vi "wd_create (WFM).vi"(7 "WFM":waveform(dbl), 8 "error in (no error)":errorcluster, 9 "data type":T1, 11 "meta in":T2={"TargetFile"=path "", "StreamMode"=enum."File", "Append?"=FALSE, "ChunkSize"=0, "TimeColumnMode"=enum."Empty", "TimestampFormat"="", "AbsoluteTime?"=FALSE, "FileAttribute "={"Creator"="", "Title"="", "SheetName"=""}, "Column"=[], "FileRef"=refnum, "MemoryRef"=[], "RecordInfo"=[], " ChannelPreviousInfo"=[], "ChannelFirstRecord"=[], "PredefinedFormattedValueLength"=20, "DiskTemplate"={"XMLRef"=[refnum, refnum, refnum, refnum, refnum, refnum], "ZipPath"=path "", "MetaFile"={"Ref"=refnum, "NextRow"=0, "NextPosition"=0, "Block"=[]}, "TempFolder"=path ""}}) -> (0 "error out":errorcluster, 3 "meta out":T2={"TargetFile"=path "", "StreamMode"=enum."File", "Append?"=FALSE, "ChunkSize"=0, "TimeColumnMode"=enum."Empty", "TimestampFormat"="", "AbsoluteTime?"=FALSE, "FileAttribute "={"Creator"="", "Title"="", "SheetName"=""}, "Column"=[], "FileRef"=refnum, "MemoryRef"=[], "RecordInfo"=[], " ChannelPreviousInfo"=[], "ChannelFirstRecord"=[], "PredefinedFormattedValueLength"=20, "DiskTemplate"={"XMLRef"=[refnum, refnum, refnum, refnum, refnum, refnum], "ZipPath"=path "", "MetaFile"={"Ref"=refnum, "NextRow"=0, "NextPosition"=0, "Block"=[]}, "TempFolder"=path ""}})   [LabVIEW 2020, in "NI_ExcelFile.lvlib"]
uses:
  <vilib>/express/express shared/NI_ExcelFile/NI_ExcelFile.lvlib
  <vilib>/express/express shared/NI_ExcelFile/Ctrls/MainData.ctl
  <vilib>/express/express shared/NI_ExcelFile/Ctrls/StreamMode.ctl
  <vilib>/express/express shared/NI_ExcelFile/Ctrls/TimeColumnMode.ctl
  <vilib>/express/express shared/NI_ExcelFile/Ctrls/FileAttribute.ctl
  <vilib>/express/express shared/NI_ExcelFile/Ctrls/Columns.ctl
  <vilib>/express/express shared/NI_ExcelFile/Ctrls/ColumnInfo.ctl
  <vilib>/express/express shared/NI_ExcelFile/Ctrls/DataType.ctl
  <vilib>/express/express shared/NI_ExcelFile/Ctrls/wd_recordInfo.ctl
  <vilib>/express/express shared/NI_ExcelFile/Ctrls/disk_TemplateFile.ctl
  <vilib>/express/express shared/NI_ExcelFile/Ctrls/meta_file.ctl
  <vilib>/express/express shared/NI_ExcelFile/Ctrls/meta_Block.ctl
  <vilib>/express/express shared/NI_ExcelFile/Ctrls/meta_BlockType.ctl
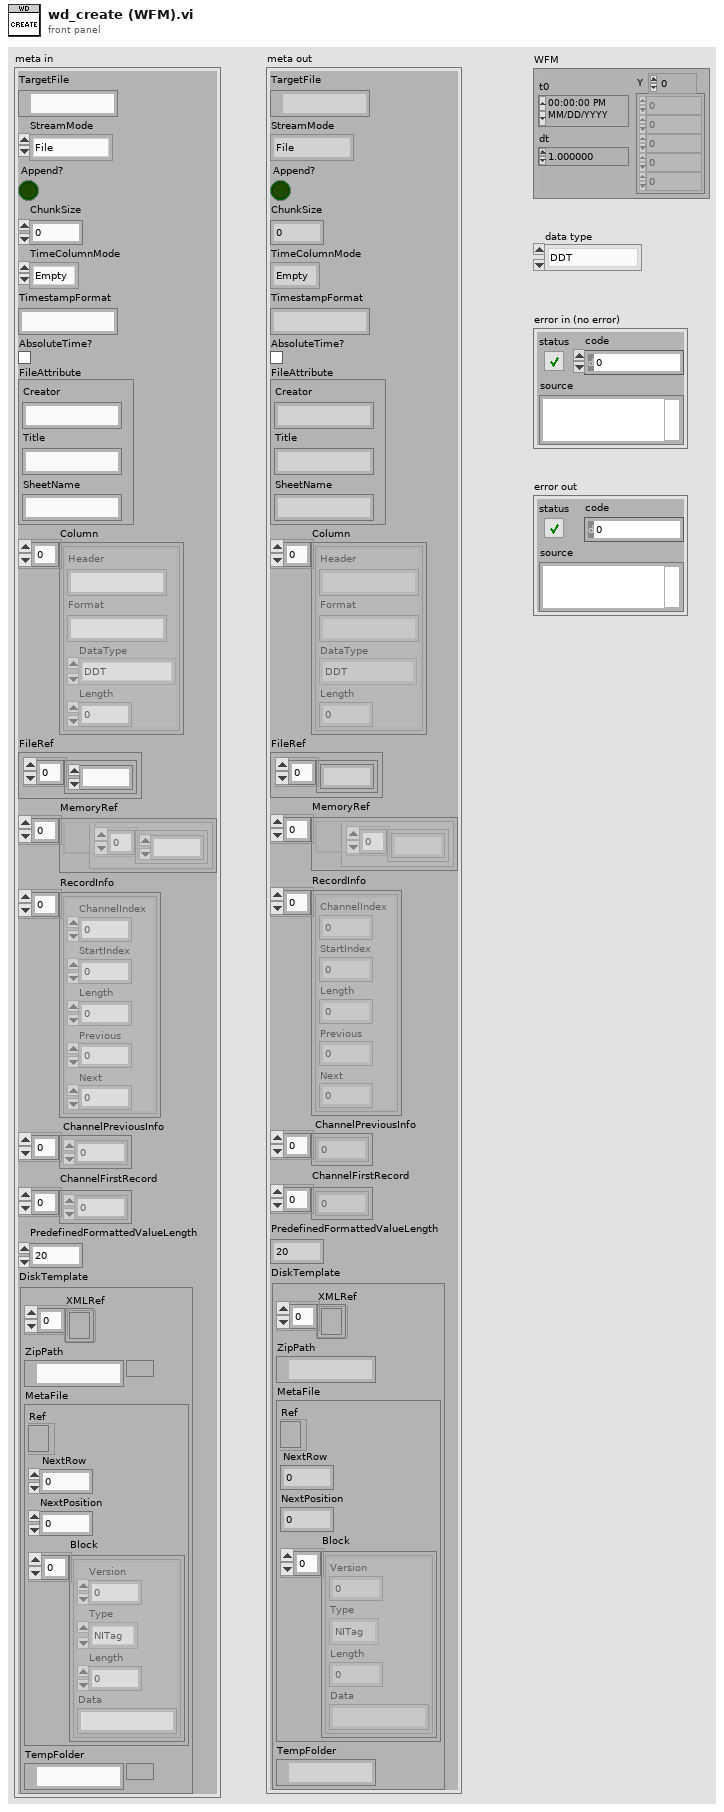
[diagram p1: front panel]
types:
  T1 = typedef "NI_ExcelFile.lvlib/DataType.ctl" = enum16{"DDT", "WFM", "Array of STR", "Array of DBL", "Array of I8", "Array of I16", "Array of I32", "Array of I64", "Array of SGL", "Array of U8", "Array of U16", "Array of U32", "Array of U64", "Array of Time"}
  T2 = typedef "NI_ExcelFile.lvlib/MainData.ctl" = cluster{"TargetFile":path, "StreamMode":T3, "Append?":bool, "ChunkSize":u64, "TimeColumnMode":T4, "TimestampFormat":string, "AbsoluteTime?":bool, "FileAttribute ":T5, "Column":T6, "FileRef":refnum<k1>, "MemoryRef":refnum<data-value>[], "RecordInfo":T8[], " ChannelPreviousInfo":u32[], "ChannelFirstRecord":u32[], "PredefinedFormattedValueLength":i64, "DiskTemplate":T9}
  T3 = typedef "NI_ExcelFile.lvlib/StreamMode.ctl" = enum16{"File", "Memory"}
  T4 = typedef "NI_ExcelFile.lvlib/TimeColumnMode.ctl" = enum16{"Empty", "OnePerCh", "One"}
  T5 = typedef "NI_ExcelFile.lvlib/FileAttribute.ctl" = cluster{"Creator":string, "Title":string, "SheetName":string}
  T6 = typedef "NI_ExcelFile.lvlib/Columns.ctl" = T7[]
  T7 = typedef "NI_ExcelFile.lvlib/ColumnInfo.ctl" = cluster{"Header":string, "Format":string, "DataType":T1, "Length":u64}
  T8 = typedef "NI_ExcelFile.lvlib/wd_recordInfo.ctl" = cluster{"ChannelIndex":u32, "StartIndex":u64, "Length":u64, "Previous":i32, "Next":i32}
  T9 = typedef "NI_ExcelFile.lvlib/disk_TemplateFile.ctl" = cluster{"XMLRef":refnum<file>[], "ZipPath":path, "MetaFile":T10, "TempFolder":path}
  T10 = typedef "NI_ExcelFile.lvlib/meta_file.ctl" = cluster{"Ref":refnum<file>, "NextRow":i32, "NextPosition":i64, "Block":T11[]}
  T11 = typedef "NI_ExcelFile.lvlib/meta_Block.ctl" = cluster{"Version":u16, "Type":T12, "Length":i32, "Data":string}
  T12 = typedef "NI_ExcelFile.lvlib/meta_BlockType.ctl" = enum16{"NITag", "File", "Column"}
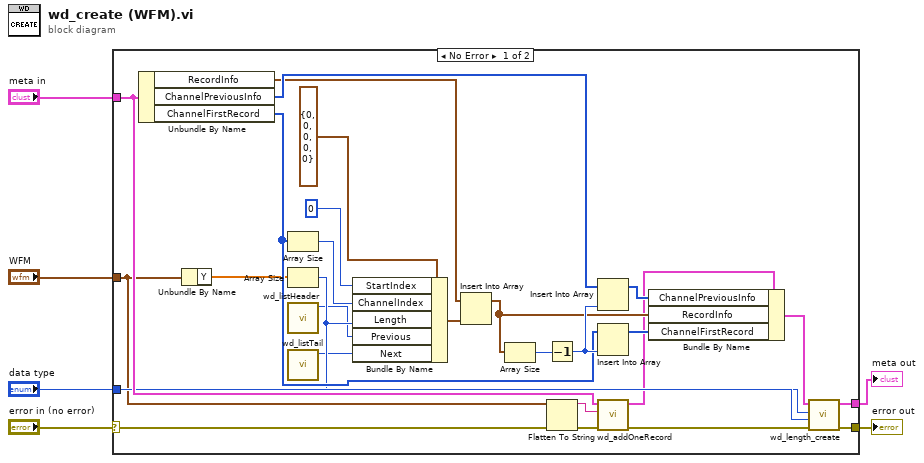
[diagram p0: block diagram]
diagram:
  n1 = case shown="No Error" "error in (no error)" {
    selector: "error in (no error)" -> [w24 w34]
    tunnel: "data type" -> [w21 _]
    tunnel: [w18 w35] -> w5
    tunnel: "meta in" -> [w22 w35]
    tunnel: [w16 w34] -> w2
    tunnel: "WFM" -> [w7 _]
    frame No Error {
      n2 = Unbundle By Name(w22) -> ("RecordInfo"=w27:T8[], "ChannelPreviousInfo"=w28:u32[], "ChannelFirstRecord"=w26:u32[])
      n3 = Unbundle By Name(w7) -> ("Y"=w8:dbl[])
      n4 = Array Size(array=w26) -> (size(s)=w11:i32)
      n5 = Array Size(array=w8) -> (size(s)=w13:i32)
      n6 = call <vilib>:"wd_listHeader.vi"() -> ("list header"=w10:i32)  [unwired: 11 in]
      n7 = call <vilib>:"wd_listTail.vi"() -> ("list tail"=w9:i32)  [unwired: 11 in]
      n8 = Bundle By Name(cluster=T8 {"ChannelIndex"=0, "StartIndex"=0, "Length"=0, "Previous"=0, "Next"=0} ("Channel Info"), "StartIndex"=u64 0 ("Start Index"), "ChannelIndex"=w11, "Length"=w13, "Previous"=w10, "Next"=w9) -> (w14:T8)
      n9 = Insert Into Array(array=w27, new element=w14) -> (w31:T8[])  [unwired: 1 in]
      n10 = Array Size(array=w31) -> (size(s)=w30:i32)
      n11 = Decrement(x=w30) -> (x-1=w32:i32)
      n12 = Flatten To String(anything=w7, error in (no error)=w24) -> (data string=w25:string, error out=w23:errorcluster)  [unwired: 2 in, 1 out]
      n13 = Insert Into Array(array=w28, new element=w32) -> (w29:u32[])  [unwired: 1 in]
      n14 = Insert Into Array(array=w26, new element=w32) -> (w33:u32[])  [unwired: 1 in]
      n15 = call <vilib>:"wd_addOneRecord.vi"("error in (no error)"=w23, "data"=w25, "meta in"=w22) -> ("error out"=w17:errorcluster, "meta out"=w20:T2)  [unwired: 7 in]
      n16 = Bundle By Name(cluster=w20, "ChannelPreviousInfo"=w29, "RecordInfo"=w31, "ChannelFirstRecord"=w33) -> (w19:T2)
      n17 = call <vilib>:"wd_length_create.vi"("error in (no error)"=w17, "data type"=w21, "size"=w13, "meta in"=w19) -> ("error out"=w16:errorcluster, "meta out"=w18:T2)  [unwired: 6 in]
    }
    frame Error {
    }
  }
  "error out" <- w2
  "meta out" <- w5
